vi "Host_8840.vi"() -> ()   [LabVIEW 2019]
panel:
  in  "stop":bool
  out "FH:Vsup Present":bool
  in  "HF:Motor":bool=TRUE
  out "GH:Current Sense":i32
  out "FH:DriveStatus":i32
  out "FH:DriveFa":bool
  in  "HG:Drive Direction":i16
  in  "HF:Enable E-Stop":bool
  out "Waveform Chart":i32(graph)
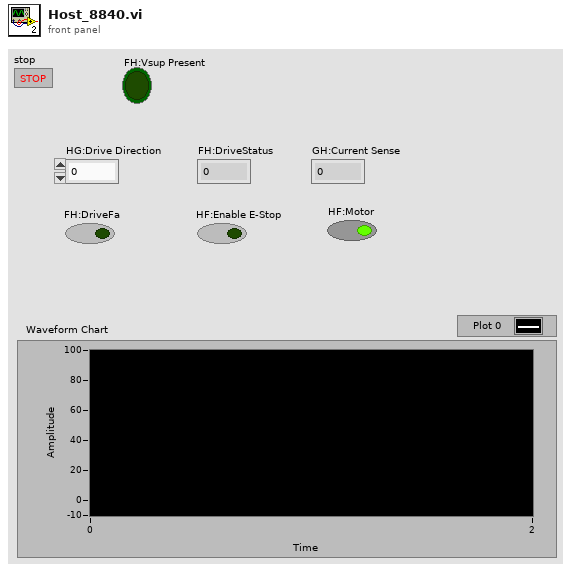
[diagram p1: front panel]
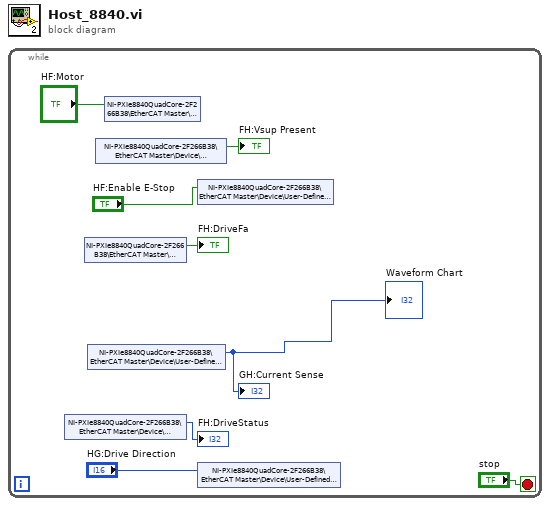
[diagram p0: block diagram]
diagram:
  n1 = while {
    stop <- "stop" stop-if-true
    n2 = shared-variable "NI-PXIe8840QuadCore-2F266B38\\EtherCAT Master\\Device\\User-Defined Variables\\FH:DriveStatus"() -> (→"FH:DriveStatus":i32)  [unwired: 1 in, 1 out]
    n3 = shared-variable "NI-PXIe8840QuadCore-2F266B38\\EtherCAT Master\\Device\\User-Defined Variables\\FH:DriveFa"() -> (→"FH:DriveFa":bool)  [unwired: 1 in, 1 out]
    n4 = shared-variable "NI-PXIe8840QuadCore-2F266B38\\EtherCAT Master\\Device\\User-Defined Variables\\GH:Current Sense"() -> (→"GH:Current Sense" →"Waveform Chart":i32)  [unwired: 1 in, 1 out]
    n5 = shared-variable "NI-PXIe8840QuadCore-2F266B38\\EtherCAT Master\\Device\\User-Defined Variables\\FH:Vsup Present"() -> (→"FH:Vsup Present":bool)  [unwired: 1 in, 1 out]
    n6 = shared-variable "NI-PXIe8840QuadCore-2F266B38\\EtherCAT Master\\Device\\User-Defined Variables\\HF:Motor"("HF:Motor") -> ()  [unwired: 1 in, 1 out]
    n7 = shared-variable "NI-PXIe8840QuadCore-2F266B38\\EtherCAT Master\\Device\\User-Defined Variables\\HF:Enable E-Stop"("HF:Enable E-Stop") -> ()  [unwired: 1 in, 1 out]
    n8 = shared-variable "NI-PXIe8840QuadCore-2F266B38\\EtherCAT Master\\Device\\User-Defined Variables\\HG:Drive Direction"("HG:Drive Direction") -> ()  [unwired: 1 in, 1 out]
  }
